vi "Get Property Parameters Configuration File Required.vi"(8 "error in":errorcluster, 11 "configuration files ref":T1 format="%.0x") -> (0 "error out":errorcluster, 2 "required":bool, 3 "configuration files ref out":T1 format="%.0x", 4 "found?":bool)   [LabVIEW 2020, in "Ballard MIL-STD-1553 Scripting.lvlib"]
uses:
  <vilib>/NI VeriStand/Custom Device API/Custom Device Item Ref.ctl
  Constants.vi
  Ballard MIL-STD-1553 Scripting.lvlib
  <vilib>/NI VeriStand/Custom Device API/Custom Device API.lvlib
  <vilib>/NI VeriStand/Custom Device API/Get Item Property (Boolean).vi
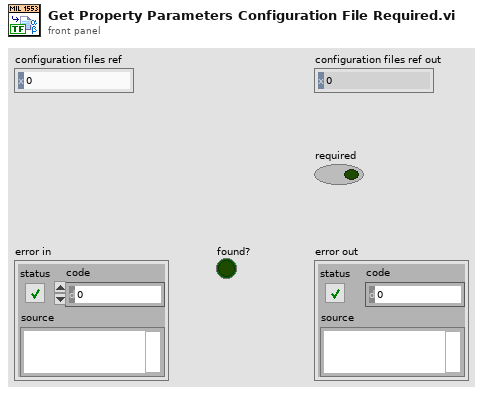
[diagram p1: front panel]
types:
  T1 = typedef "Custom Device API.lvlib/Custom Device Item Ref.ctl" = u64
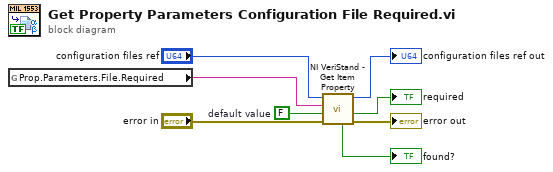
[diagram p0: block diagram]
diagram:
  w3 = FALSE  # default value
  n1 = global read "Constants.vi" "Prop.Parameters.File.Required"() -> (w4:string)
  n2 = call-poly <vilib>:"NI VeriStand - Get Item Property.vi"("error in (no error)"="error in", "Default Value"=w3, "Property Name"=w4, "Item Ref in"="configuration files ref") -> ("error out"=→"error out":errorcluster, "Value"=→"required":bool, "Item Ref out"=→"configuration files ref out":T1, "Found?"=→"found?":bool)  [unwired: 4 in]
